vi "PID_velocity_radian.vi"() -> ()   [LabVIEW 2014]
uses:
  <vilib>/FPGAPlugInAG/cRIO-9068/niLvFpga_Open_cRIO-9068.vi
  <vilib>/rvi/interface/common/dynamic/niFpgaDynamicAddResources.vi
  <vilib>/Utility/error.llb/Error Cluster From Error Code.vi
  <vilib>/rvi/errors/niLvFpgaAdjustHostInterfaceError.vi
  <vilib>/addons/control/pid/pid.llb/PID (DBL).vi
  <vilib>/FPGAPlugInAG/Dynamic/niLvFpga_Close_Dynamic.vi
  <vilib>/rvi/interface/nirviOpenFPGA/nirviOpenFPGA.xnode
  FPGA Bitfiles/Motortest_FPGATarget_test6auto_Jx62XASY7Q8.lvbitx
  <vilib>/rvi/interface/nirviReadWriteControl/nirviReadWriteControl.xnode
  <vilib>/rvi/interface/nirviCloseFPGA/nirviCloseFPGA.xnode
  NiFpgaLv.dll
  <vilib>/rvi/interface/Simulation/niFpgaSimulationCallBeginRW.vi
  <vilib>/addons/control/pid/NI_PID_pid.lvlib
panel:
  out "Duty Cycle":cluster{dbl[], dbl[]}(graph)
  out "Velocity":cluster{dbl[], sgl[]}(graph)
  out "Duty Cycle":dbl(slide)=0.3041260266125599 scale=0.0..1.0
  out "Error":dbl(slide)=-0.0220947265625 scale=0.0..200.0
  in  "output range":cluster{"output high":dbl, "output low":dbl}={"output high"=1.0, "output low"=-1.0} {"output low" format="%.2f"; "output high" format="%.2f"}
  in  "PID gains":T1={"proportional gain (Kc)"=0.0006, "integral time (Ti, min)"=0.0005, "derivative time (Td, min)"=0.0} {"derivative time (Td, min)" format="%.4f"; "integral time (Ti, min)" format="%.4e"; "proportional gain (Kc)" format="%.4e"}
  in  "Desired Velocity":dbl=300.0 format="%.2f"
  out "Velocity":sgl=300.0221
  out "Position":sgl=1200.7482
  in  "stop":bool
  # "Kp = 1E-3\nKi = 5E-4"
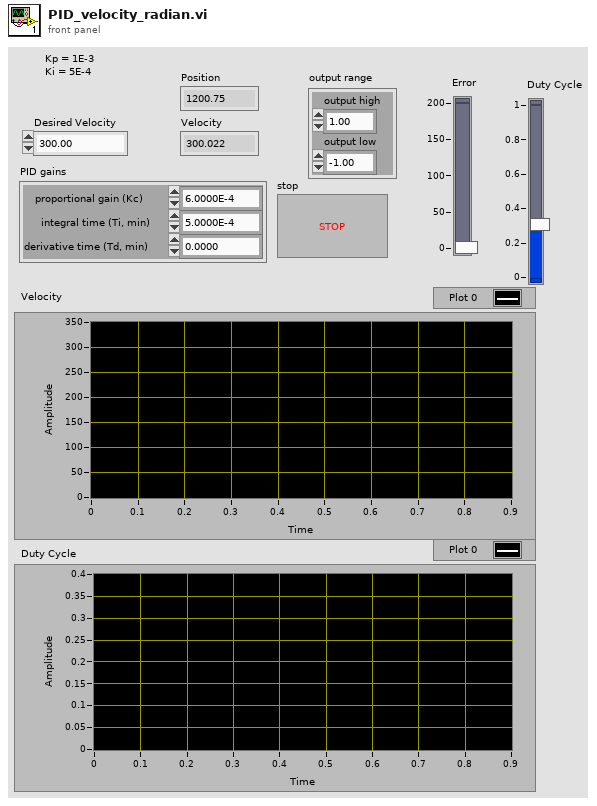
[diagram p1: front panel]
types:
  T1 = cluster{"proportional gain (Kc)":dbl, "integral time (Ti, min)":dbl, "derivative time (Td, min)":dbl}
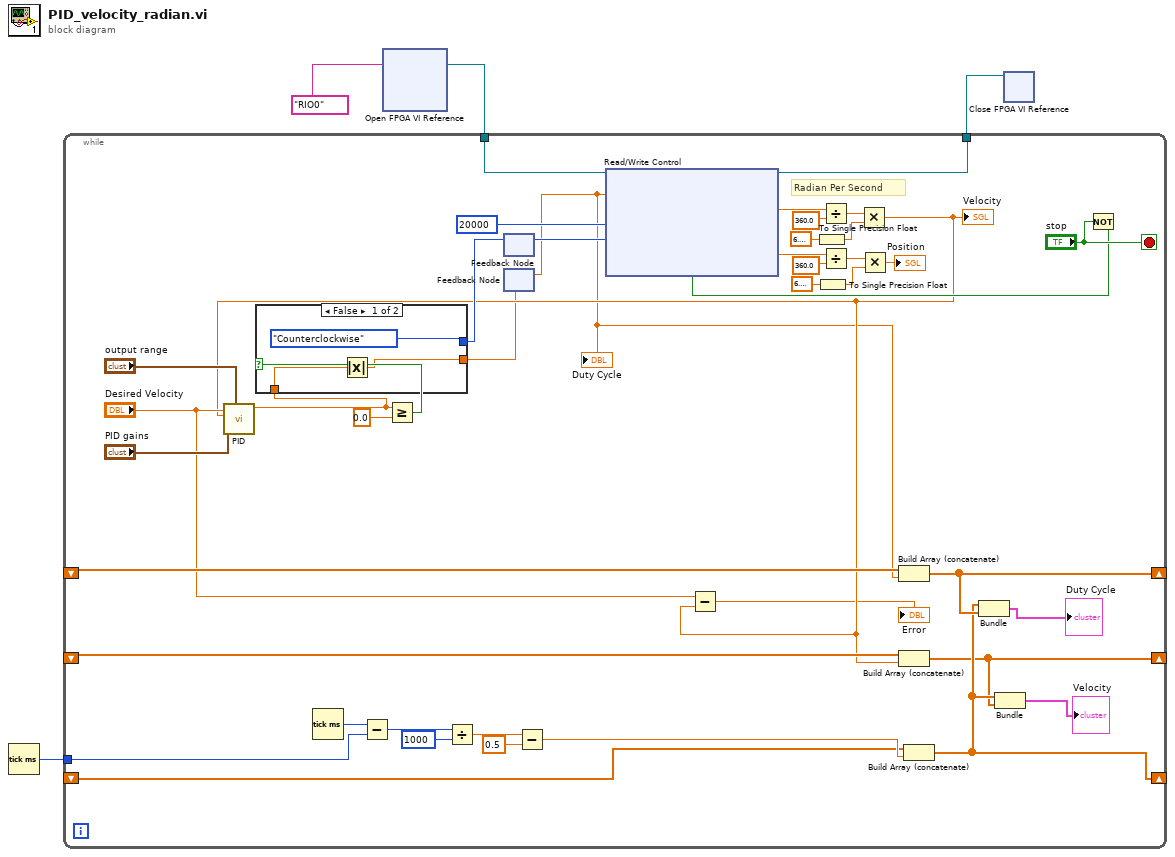
[diagram p0: block diagram]
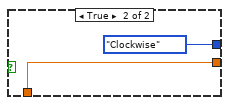
[diagram p2: hidden frame]
diagram:
  n1 = Tick Count (ms)() -> (millisecond timer value=w1:u32)
  n2 = xnode "Open FPGA VI Reference"("resource name"=tag "RIO0") -> ("FPGA VI Reference Out"=w2:refnum<k20>)  [unwired: 1 in, 1 out]
  n3 = while {
    tunnel: w2 -> [w47]
    tunnel: [w46] -> w4
    shift-right: [w9] -> _
    shift-left: _ -> [w40]
    shift-right: [w6] -> _
    shift-left: _ -> [w39]
    tunnel: w1 -> [w13]
    shift-right: [w7] -> _
    shift-left: _ -> [w10]
    stop <- "stop" stop-if-true
    # "Radian Per Second"
    n4 = Tick Count (ms)() -> (millisecond timer value=w16:u32)
    n5 = Subtract(x=w16, y=w13) -> (x-y=w12:u32)
    n6 = Divide(x=w12, y=u32 1000) -> (x/y=w15:dbl)
    n7 = feedback #1() -> (w32:enum8{"Clockwise", "Counterclockwise"})  [unwired: 1 in]
    n8 = feedback #2() -> (w18:dbl)  [unwired: 1 in]
    "Duty Cycle" <- w18
    n9 = Subtract(x=w15, y=0.5) -> (x-y=w11:dbl)
    n10 = To Single Precision Float(number=6.283185307179586 ("Pi Multiplied By 2")) -> (single precision float=w28:sgl)
    n11 = To Single Precision Float(number=6.283185307179586 ("Pi Multiplied By 2")) -> (single precision float=w26:sgl)
    n12 = Build Array (concatenate)(w40, w18) -> (w9:dbl[])
    n13 = Build Array (concatenate)(w10, w11) -> (w7:dbl[])
    n14 = Bundle(w7, w9) -> (→"Duty Cycle":cluster{dbl[], dbl[]})  [unwired: 1 in]
    n15 = Not(x="stop") -> (.not. x?=w44:bool)
    n16 = xnode "Read/Write Control"("FPGA VI Reference In"=w47, "duty cycle (periods)"=w18, "Velocity Interval (uSec)"=u32 20000, "Mod1/Drive Direction"=w32, "Mod1/Motor"=w44) -> ("FPGA VI Reference Out"=w46:refnum<k20>, "Velocity (Degrees/Second)"=w37:sgl, "Position (Degrees)"=w22:sgl)  [unwired: 1 in, 1 out]
    n17 = Divide(x=w37, y=sgl 360.0) -> (x/y=w29:sgl)
    n18 = Divide(x=w22, y=sgl 360.0) -> (x/y=w25:sgl)
    n19 = Multiply(x=w29, y=w28) -> (x*y=w27:sgl)
    "Velocity" <- w27
    n20 = call-poly <vilib>:"PID.vi"("output range"="output range", "PID gains"="PID gains", "process variable"=w27, "setpoint"="Desired Velocity") -> ("output"=w34:dbl)  [unwired: 6 in, 1 out]
    n21 = Greater Or Equal?(x=w34, y=0.0) -> (x >= y?=w35:bool)
    n22 = case shown="False" w35 {
      tunnel: w34 -> [w48 w52]
      tunnel: [w49 w52] -> w19
      tunnel: [enum8{"Clockwise", "Counterclockwise"}."Counterclockwise" ("Mod1/Drive Direction") enum8{"Clockwise", "Counterclockwise"}."Clockwise" ("Mod1/Drive Direction")] -> w33
      frame False {
        n23 = Absolute Value(x=w48) -> (abs(x)=w49:dbl)
      }
      frame True {
      }
    }
    n24 = feedback-in #1(w33) -> ()
    n25 = feedback-in #2(w19) -> ()
    n26 = Subtract(x="Desired Velocity", y=w27) -> (x-y=→"Error":dbl)
    n27 = Multiply(x=w25, y=w26) -> (x*y=→"Position":sgl)
    n28 = Build Array (concatenate)(w39, w27) -> (w6:sgl[])
    n29 = Bundle(w7, w6) -> (→"Velocity":cluster{dbl[], sgl[]})  [unwired: 1 in]
  }
  n30 = xnode "Close FPGA VI Reference"("FPGA VI Reference In"=w4) -> ()  [unwired: 1 in, 1 out]
